vi "GetStationFullName.vi"(8 "error in":errorcluster, 11 "OperationRun in":refnum<class "OperationRun.lvclass">) -> (0 "error out":errorcluster, 2 "StationFullName":string, 3 "OperationRun out":refnum<class "OperationRun.lvclass">)   [LabVIEW 2021, in "ProligentXMLGenerator.lvlib" / "OperationRun.lvclass"]
doc: "Defines the station where the operation run was executed.\n\nThis attribute cannot be updated."
uses:
  OperationRun.lvclass
  OperationRun.lvclass/OperationRun.ctl
  Base/Attribute/Attribute.lvclass
  Base/FullName/FullName.lvclass
  C:/Projects/proligent-xml-generator-labview/src/ProligentXMLGenerator/Base/NonEmptyString/NonEmptyString.lvclass
  C:/Projects/proligent-xml-generator-labview/src/ProligentXMLGenerator/Base/String/String.lvclass
  C:/Projects/proligent-xml-generator-labview/src/ProligentXMLGenerator/Base/Attribute/Attribute.lvclass
  C:/Projects/proligent-xml-generator-labview/src/ProligentXMLGenerator/Base/FullName/FullName.lvclass
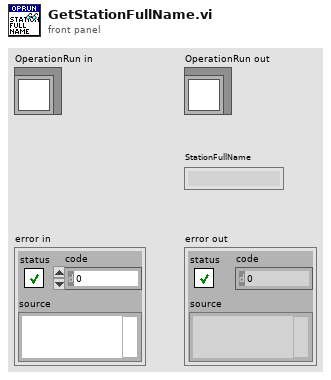
[diagram p1: front panel]
types:
  T1 = typedef "ProligentXMLGenerator.lvlib/OperationRun.lvclass/Data.ctl" = cluster{"Name":string, "Characteristics":refnum<class "Characteristic.lvclass">[], "Documents":refnum<class "Document.lvclass">[], "SequenceRuns":refnum<class "SequenceRun.lvclass">[], "FailureReferences":refnum<class "FailureReference.lvclass">[], "SequenceRunReferences":refnum<class "SequenceRunReference.lvclass">[], "CustomData":refnum<class "CustomData.lvclass">, "OperationRunId":refnum<class "Guid.lvclass">, "ProcessFullName":refnum<class "ProcessFullName.lvclass">, "ProcessVersion":refnum<class "NonEmptyString_64.lvclass">, "OperationName":refnum<class "NonEmptyString_65.lvclass">, "StationFullName":refnum<class "FullName.lvclass">, "User":refnum<class "NonEmptyString_255.lvclass">, "CallingOperationRunId":refnum<class "Guid.lvclass">, "OperationStatus":refnum<class "ExecutionStatus.lvclass">, "OperationRunStartTime":refnum<class "DateTime.lvclass">, "OperationRunEndTime":refnum<class "DateTime.lvclass">, "TimeZoneInfoId":string}
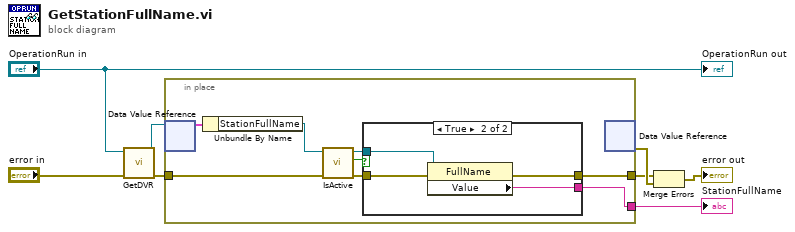
[diagram p0: block diagram]
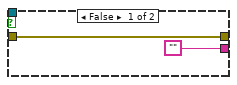
[diagram p2: hidden frame]
diagram:
  n1 = call "GetDVR.vi"("error in"="error in", "OperationRun"="OperationRun in") -> ("error out"=w3:errorcluster, "DVRReference"=w2:refnum<data-value>)  [unwired: 8 in]
  n2 = in-place "In Place Element Structure" {
    in-place-border: [w15] -> w7
    in-place-border: w3 -> [w12]
    in-place-border: [w14] -> w5
    n3 = in-place-dvr #1(w2) -> (w16:T1)  [unwired: 1 out]
    n4 = Unbundle By Name(w16) -> ("StationFullName"=w11:refnum<class "FullName.lvclass">)
    n5 = call "IsActive.vi"("error in"=w12, "Attribute in"=w11) -> ("error out"=w13:errorcluster, "IsActive"=w9:bool, "Attribute in"=w10:refnum<class "FullName.lvclass">)  [unwired: 7 in]
    n6 = case shown="True" w9 {
      tunnel: ["" ("Empty String Constant") w22] -> w15
      tunnel: [w17 w21] -> w14
      tunnel: w13 -> [w17 w20]
      tunnel: w10 -> [_ w19]
      frame False {
      }
      frame True {
        n7 = property on="Property Node" class="FullName"(reference=w19, error in=w20) -> (error out=w21:errorcluster, "Value"=w22:string)  [unwired: 1 out]
      }
    }
    n8 = in-place-dvr #1() -> (w8:errorcluster)  [unwired: 1 in, 1 out]
  }
  "StationFullName" <- w7
  n9 = Merge Errors(w5, w8) -> (→"error out":errorcluster)
  "OperationRun out" <- "OperationRun in"
